vi "Hide Animated Busy Icon with Message.vi"(4 "Animated Busy Icon Control Name (Animated Busy Icon)":string="Animated Busy Icon", 5 "Already active? (F)":bool, 6 "Message Control Name (Message)":string="Message", 7 "Message":string, 9 "Error In":errorcluster, 11 "Target VI reference":refnum<vi>) -> (1 "Error Out":errorcluster)   [LabVIEW 2019]
doc: "This VI passes error in through and ignores it"
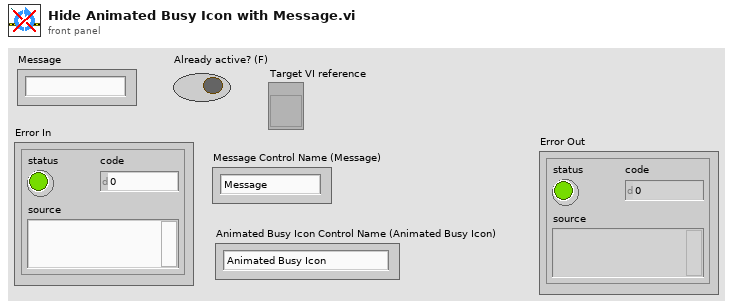
[diagram p1: front panel]
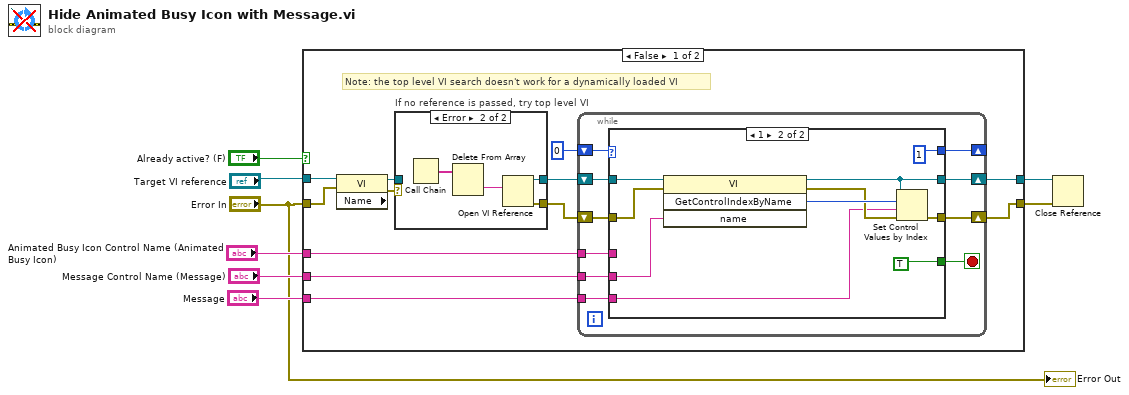
[diagram p0: block diagram]
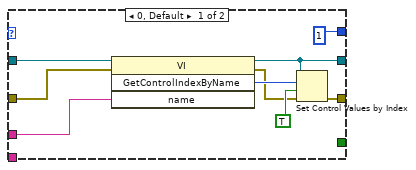
[diagram p3: hidden frame]
diagram:
  n1 = case shown="False" "Already active? (F)" {
    tunnel: [w20 w57] -> w8
    tunnel: [w19 w56] -> w7
    tunnel: "Message Control Name (Message)" -> [w17 _]
    tunnel: "Animated Busy Icon Control Name (Animated Busy Icon)" -> [w16 _]
    tunnel: "Message" -> [w15 _]
    tunnel: "Target VI reference" -> [w12 w57]
    tunnel: "Error In" -> [w9 w56]
    frame False {
      # "Note: the top level VI search doesn't work for a dynamically loaded VI"
      n2 = property class="VI" props=["Name"](reference=w12, error in=w9) -> (reference out=w11:refnum<vi>, error out=w10:errorcluster)  [unwired: 1 out]
      n3 = case "If no reference is passed, try top level VI" shown="Error" w10 {
        selector: w10 -> [w21 _]
        tunnel: [w21 w26] -> w13
        tunnel: [w22 w25] -> w14
        tunnel: w11 -> [w22 _]
        frame No Error {
        }
        frame Error {
          n4 = Call Chain() -> (call chain=w23:string[])
          n5 = Delete From Array(array=w23) -> (deleted portion=w24:string)  [unwired: 2 in, 1 out]
          n6 = Open VI Reference(vi path=w24) -> (vi reference=w25:refnum<vi>, error out=w26:errorcluster)  [unwired: 5 in]
        }
      }
      n7 = while {
        shift-right: [w33] -> w19
        shift-left: w13 -> [w36]
        shift-right: [w34] -> w20
        shift-left: w14 -> [w35]
        shift-right: [w31] -> _
        shift-left: 0 -> [w32]
        tunnel: w17 -> [w29]
        tunnel: w16 -> [w28]
        tunnel: w15 -> [w27]
        stop <- w30 stop-if-true
        n8 = case shown="1" w32 {
          tunnel: w36 -> [w42 w53]
          tunnel: w35 -> [w41 w52]
          tunnel: [w40 w51] -> w34
          tunnel: [w39 w50] -> w33
          tunnel: [1 1] -> w31
          tunnel: [_ TRUE] -> w30
          tunnel: w29 -> [_ w47]
          tunnel: w28 -> [w37 _]
          tunnel: w27 -> [_ w46]
          frame 0, Default {
            n9 = invoke class="VI" method="GetControlIndexByName"(reference=w41, error in=w42, "name"=w37) -> (reference out=w40:refnum<vi>, error out=w43:errorcluster, "GetControlIndexByName"=w45:i32)  [unwired: 1 in, 1 out]
            n10 = Set Control Values by Index(0:w40, 1:w45, 2:TRUE ("Visible"), 3:w43) -> (11:w39:errorcluster)
          }
          frame 1 {
            n11 = invoke class="VI" method="GetControlIndexByName"(reference=w52, error in=w53, "name"=w47) -> (reference out=w51:refnum<vi>, error out=w54:errorcluster, "GetControlIndexByName"=w55:i32)  [unwired: 1 in, 1 out]
            n12 = Set Control Values by Index(0:w51, 1:w55, 2:w46, 3:w54) -> (11:w50:errorcluster)
          }
        }
      }
    }
    frame True {
    }
  }
  n13 = Close Reference(reference=w8, error in (no error)=w7) -> ()  [unwired: 1 out]
  "Error Out" <- "Error In"
